vi "Set Channel.vi"(6 "timeout (ms)":i32, 8 "newVal":dbl, 9 "name":string, 10 "Gateway IP Address (\"\": localhost)":string, 11 "Sequence Context":refnum<k7>) -> (0 "error out":errorcluster, 1 "timed out?":bool, 2 "Report Text":string)   [LabVIEW 2014, in "Set Channels.lvlib"]
uses:
  Set Channels.lvlib
  <vilib>/NI Veristand/Execution/Workspace/NI VeriStand - Set Single Channel Value.vi
  <vilib>/NI Veristand/Execution/Workspace/NI VeriStand - Get Single Channel Value.vi
  <vilib>/NI Veristand/Execution/Workspace/NI_VS Workspace ExecutionAPI.lvlib
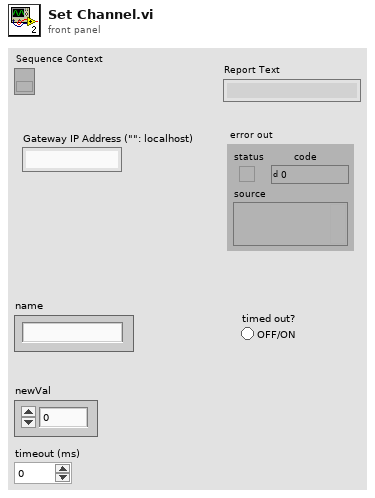
[diagram p1: front panel]
types:
  T1 = typedef "NI_VS Workspace ExecutionAPI.lvlib/WorkspaceAPI.ctl" = refnum<k24>
  T2 = typedef "TestStand - Status Monitor.ctl" = cluster{"Sequence Context":refnum<k7>, "Execution":refnum<k7>, "Termination Monitor":refnum<k7>}
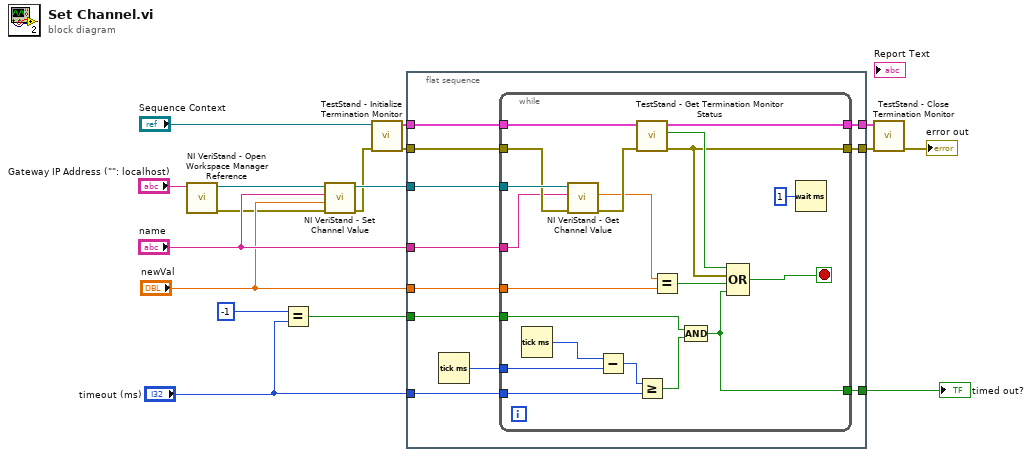
[diagram p0: block diagram]
diagram:
  n1 = call <vilib>:"NI VeriStand - Open Workspace Manager Reference.vi"("Gateway IP Address (\"\": localhost)"="Gateway IP Address (\"\": localhost)") -> ("error out"=w6:errorcluster, "WorkspaceManager"=w7:T1)  [unwired: 9 in]
  n2 = Equal?(x=-1, y="timeout (ms)") -> (x = y?=w2:bool)
  n3 = call-poly <vilib>:"NI VeriStand - Set Channel Value.vi"("error in (no error)"=w6, "Value"="newVal", "Channel"="name", "WorkspaceManager in"=w7) -> ("error out"=w13:errorcluster, "WorkspaceManager out"=w17:T1)  [unwired: 6 in]
  n4 = call <vilib>:"TestStand - Initialize Termination Monitor.vi"("error in (no error)"=w13, "Sequence Context In"="Sequence Context") -> ("error out"=w12:errorcluster, "Status Monitor Out"=w15:T2)  [unwired: 8 in]
  n5 = flat-sequence {
    tunnel: w17 -> [w28]
    tunnel: w15 -> [w27]
    tunnel: [w26] -> w14
    tunnel: w12 -> [w25]
    tunnel: "name" -> [w24]
    tunnel: "newVal" -> [w23]
    tunnel: [w22] -> w9
    tunnel: "timeout (ms)" -> [w20]
    tunnel: w2 -> [w19]
    tunnel: [w18] -> w1
    frame #0 {
      n6 = Tick Count (ms)() -> (millisecond timer value=w21:u32)
      n7 = while {
        tunnel: w28 -> [w48]
        tunnel: w27 -> [w47]
        tunnel: [w46] -> w26
        tunnel: w25 -> [w45]
        tunnel: w24 -> [w44]
        tunnel: w23 -> [w41]
        tunnel: [w37] -> w22
        tunnel: w21 -> [w34]
        tunnel: w20 -> [w32]
        tunnel: w19 -> [w30]
        tunnel: [w29] -> w18
        stop <- w39 stop-if-true
        n8 = Tick Count (ms)() -> (millisecond timer value=w35:u32)
        n9 = call-poly <vilib>:"NI VeriStand - Get Channel Value.vi"("error in (no error)"=w45, "Channel"=w44, "WorkspaceManager in"=w48) -> ("error out"=w43:errorcluster, "Value"=w42:dbl)  [unwired: 6 in, 1 out]
        n10 = Subtract(x=w35, y=w34) -> (x-y=w33:u32)
        n11 = call <vilib>:"TestStand - Get Termination Monitor Status.vi"("error in (no error)"=w43, "Status Monitor In"=w47) -> ("error out"=w37:errorcluster, "Terminating or Aborting"=w40:bool, "Status Monitor Out"=w46:T2)  [unwired: 7 in]
        n12 = Greater Or Equal?(x=w33, y=w32) -> (x >= y?=w31:bool)
        n13 = Equal?(x=w42, y=w41) -> (x = y?=w36:bool)
        n14 = Compound Arithmetic op=AND(w30, w31) -> (w29:bool)
        n15 = Compound Arithmetic op=OR(w40, w37, w36, w29) -> (w39:bool)
        n16 = Wait (ms)(milliseconds to wait=u32 1) -> ()  [unwired: 1 out]
      }
    }
  }
  n17 = call <vilib>:"TestStand - Close Termination Monitor.vi"("error in (no error)"=w9, "Status Monitor In"=w14) -> ("error out"=→"error out":errorcluster)  [unwired: 9 in]
  "timed out?" <- w1
